vi "gen_pdbm_testsys_reqst_queue.vi"(8 "error in (no error)":errorcluster) -> (0 "error IO":errorcluster, 3 "pdbm_testsys_reqst_event":refnum<queue>)   [LabVIEW 2015, in "pdbm_testsys_taskroute_inter.lvlib"]
uses:
  pdbm_testsys_taskroute_inter.lvlib
  UsrDefine/pdbm_testsys_reqst_data.ctl
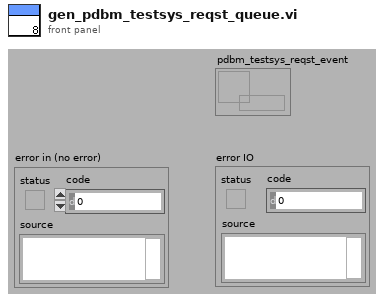
[diagram p1: front panel]
types:
  T1 = typedef "pdbm_testsys_taskroute_inter.lvlib/pdbm_testsys_reqst_data.ctl" = cluster{"TaskName":string, "Request":string, "Data":variant}
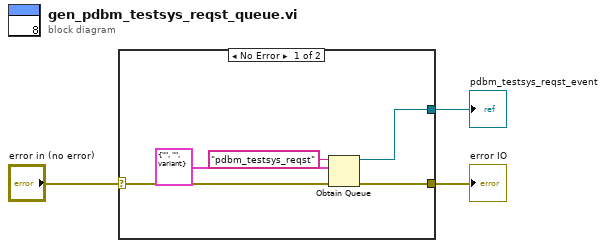
[diagram p0: block diagram]
diagram:
  n1 = case shown="No Error" "error in (no error)" {
    selector: "error in (no error)" -> [w8 w9]
    tunnel: [w5 _] -> w2
    tunnel: [w4 w9] -> w1
    frame No Error {
      n2 = Obtain Queue(name (unnamed)="pdbm_testsys_reqst", element data type=T1 {"TaskName"="", "Request"="", "Data"=variant} ("pdbm_testsys_reqst"), error in (no error)=w8) -> (queue out=w5:refnum<queue>, error out=w4:errorcluster)  [unwired: 2 in, 1 out]
    }
    frame Error {
    }
  }
  "pdbm_testsys_reqst_event" <- w2
  "error IO" <- w1
